vi "14Sheridan.vi"() -> ()   [LabVIEW 2014]
panel:
  out "Ramp Length":dbl
  in  "Ramp Angle":dbl min=0.0 max=50.0 step=0.1
  in  "Ramp Height":dbl=2.0 min=2.0 max=2.0
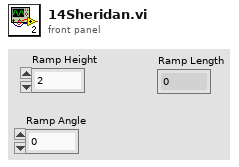
[diagram p1: front panel]
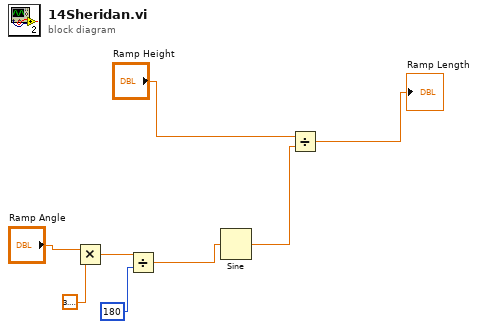
[diagram p0: block diagram]
diagram:
  n1 = Multiply(x="Ramp Angle", y=3.141592653589793) -> (x*y=w3:dbl)
  n2 = Divide(x=w3, y=180) -> (x/y=w2:dbl)
  n3 = Sine(x=w2) -> (sin(x)=w7:dbl)
  n4 = Divide(x="Ramp Height", y=w7) -> (x/y=→"Ramp Length":dbl)
